vi "SRV_Watchdog Update.vi"(0 "Watchdog local data":T1 {"System Config"."Watchdog 2 Config"."Watchdog Period (s)" format="%.3f"; "System Config"."Watchdog 2 Config"."Watchdog Command"."Value" format="%02x"; "System Config"."Watchdog 2 Config"."Watchdog Command"."Register" format="%02x"; "System Config"."Watchdog 2 Config"."Watchdog Command"."I2C Address" format="%02x"; "System Config"."Watchdog 1 Config"."Watchdog Period (s)" format="%.3f"; "System Config"."Watchdog 1 Config"."Watchdog Command"."Value" format="%02x"; "System Config"."Watchdog 1 Config"."Watchdog Command"."Register" format="%02x"; "System Config"."Watchdog 1 Config"."Watchdog Command"."I2C Address" format="%02x"}, 11 "error in (no error)":errorcluster) -> (4 "Watchdog local data out":T1 {"System Config"."Watchdog 2 Config"."Watchdog Period (s)" format="%.3f"; "System Config"."Watchdog 2 Config"."Watchdog Command"."Value" format="%02x"; "System Config"."Watchdog 2 Config"."Watchdog Command"."Register" format="%02x"; "System Config"."Watchdog 2 Config"."Watchdog Command"."I2C Address" format="%02x"; "System Config"."Watchdog 1 Config"."Watchdog Period (s)" format="%.3f"; "System Config"."Watchdog 1 Config"."Watchdog Command"."Value" format="%02x"; "System Config"."Watchdog 1 Config"."Watchdog Command"."Register" format="%02x"; "System Config"."Watchdog 1 Config"."Watchdog Command"."I2C Address" format="%02x"}, 15 "error out":errorcluster)   [LabVIEW 2009]
uses:
  SRV_Watchdog State Machine Local Data.ctl
  SubVIs/SysConfig/SRV_System Config.ctl
  SRV_Watchdog Config Cluster.ctl
  Motors/Motors Config/SRV_Motor Control Command Config.ctl
panel:
  # "I2C Address"
  # "Register"
  # "Value"
  # "Active"
  # "I2C Address"
  # "Register"
  # "Value"
  # "Active"
  # "I2C Address"
  # "Register"
  # "Value"
  # "Active"
  # "I2C Address"
  # "Register"
  # "Value"
  # "Active"
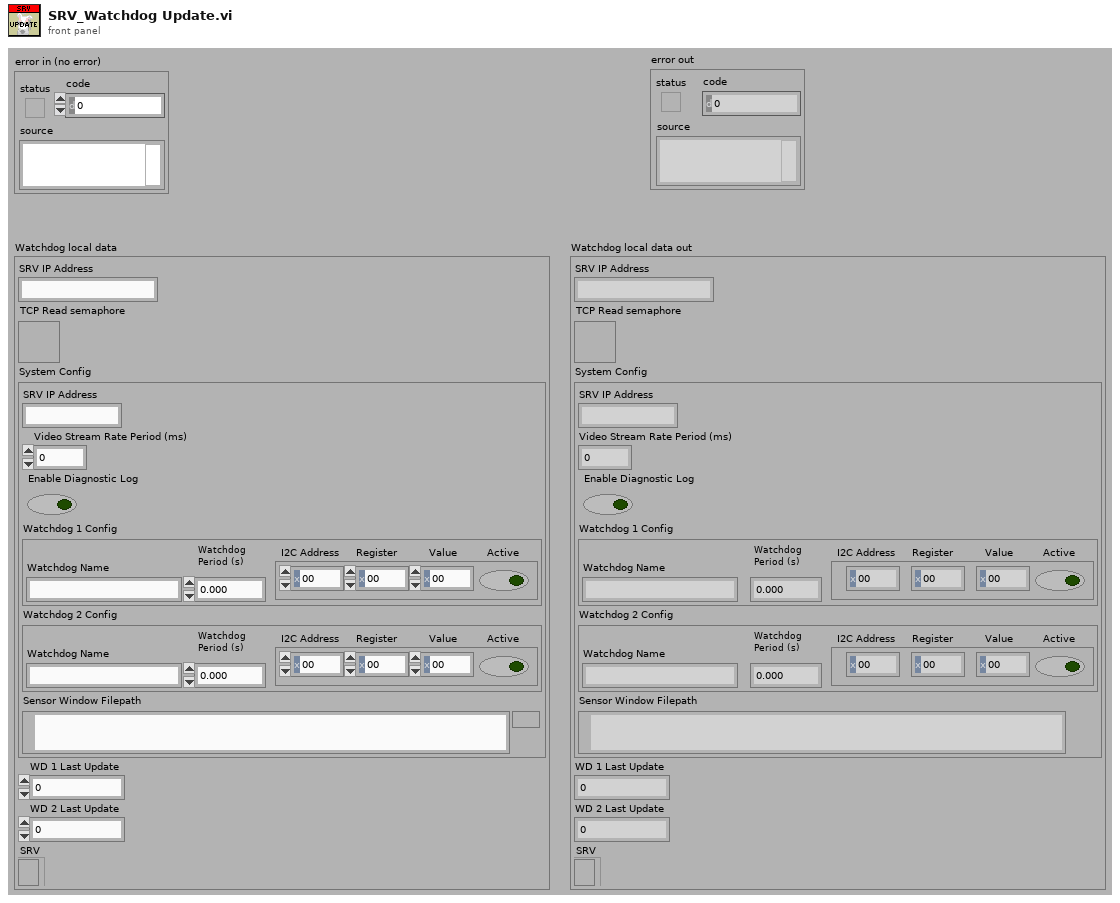
[diagram p1: front panel]
types:
  T1 = typedef "SRV_Watchdog State Machine Local Data.ctl" = cluster{"SRV IP Address":string, "TCP Read semaphore":T2, "System Config":T3, "WD 1 Last Update":dbl, "WD 2 Last Update":dbl, "SRV":refnum<k5>}
  T2 = typedef "Semaphore RefNum" = refnum<k1>
  T3 = typedef "SRV_System Config.ctl" = cluster{"SRV IP Address":string, "Video Stream Rate Period (ms)":u32, "Enable Diagnostic Log":bool, "Watchdog 1 Config":T4, "Watchdog 2 Config":T4, "Sensor Window Filepath":path}
  T4 = typedef "SRV_Watchdog Config Cluster.ctl" = cluster{"Watchdog Name":string, "Watchdog Period (s)":dbl, "Watchdog Command":T5}
  T5 = typedef "SRV_Motor Control Command Config.ctl" = cluster{"I2C Address":u8, "Register":u8, "Value":u8, "Active":bool}
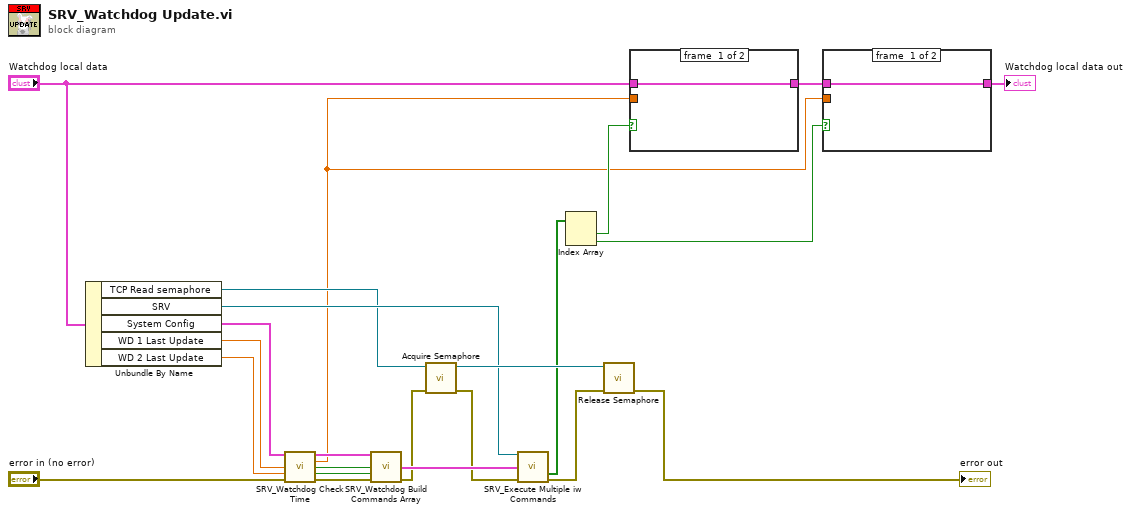
[diagram p0: block diagram]
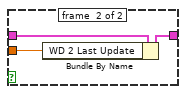
[diagram p2: hidden frame]
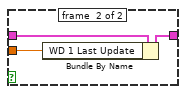
[diagram p3: hidden frame]
diagram:
  n1 = Unbundle By Name("Watchdog local data") -> ("TCP Read semaphore"=w13:T2, "SRV"=w14:refnum<k5>, "System Config"=w20:T3, "WD 1 Last Update"=w21:dbl, "WD 2 Last Update"=w22:dbl)
  n2 = call "SRV_Watchdog Check Time.vi"("System Config"=w20, "WD 1 Last Update"=w21, "WD 2 Last Update"=w22, "error in (no error)"="error in (no error)") -> ("System Config dup"=w16:T3, "Current Time"=w5:dbl, "Update WD 1?"=w12:bool, "error out"=w17:errorcluster)  [unwired: 7 in, 1 out]
  n3 = call "SRV_Watchdog Build Commands Array.vi"("System Config"=w16, "Update WD 1?"=w12, "Update WD 2?"=w12, "error in (no error)"=w17) -> ("Watchdog Commands"=w15:T5[], "error out"=w2:errorcluster)  [unwired: 9 in, 1 out]
  n4 = call <vilib>:"Acquire Semaphore.vi"("error in (no error)"=w2, "semaphore"=w13) -> ("error out"=w1:errorcluster, "semaphore out"=w19:T2)  [unwired: 3 in, 1 out]
  n5 = call "SRV_Execute Multiple iw Commands.vi"("SRV"=w14, "Motor Control Commands"=w15, "error in (no error)"=w1) -> ("Active Array"=w10:bool[], "error out"=w4:errorcluster)  [unwired: 10 in, 1 out]
  n6 = Index Array(array=w10) -> (element #1=w9:bool, element #2=w7:bool)  [unwired: 2 in]
  n7 = call <vilib>:"Release Semaphore.vi"("error in (no error)"=w4, "semaphore"=w19) -> ("error out"=→"error out":errorcluster)  [unwired: 4 in, 1 out]
  n8 = case shown="True" w9 {
    tunnel: "Watchdog local data" -> [w23 w26]
    tunnel: w5 -> [_ w25]
    tunnel: [w23 w24] -> w8
    frame #0 {
    }
    frame #1 {
      n9 = Bundle By Name(cluster=w26, "WD 1 Last Update"=w25) -> (w24:T1)
    }
  }
  n10 = case shown="True" w7 {
    tunnel: w8 -> [w27 w30]
    tunnel: w5 -> [_ w29]
    tunnel: [w27 w28] -> w6
    frame #0 {
    }
    frame #1 {
      n11 = Bundle By Name(cluster=w30, "WD 2 Last Update"=w29) -> (w28:T1)
    }
  }
  "Watchdog local data out" <- w6
